vi "Chi-Squared (Non-Central) Moments.vi"(9 "d":dbl, 10 "k":i32=1) -> (0 "error":i32, 2 "variance":dbl=2.0, 3 "mean":dbl=1.0)   [LabVIEW 2014, in "NI_Gmath.lvlib"]
doc: "Returns the expected mean and variance of the random variate X, where X describes the selected distribution type. You must manually select the polymorphic instance to use."
uses:
  NI_Gmath.lvlib
  st_error_code.ctl
panel:
  # "Chi-Squared (Non-Central) Moments"
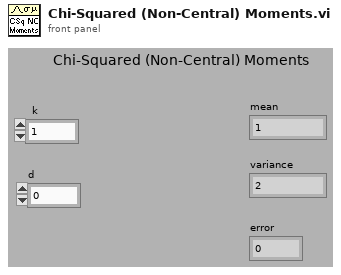
[diagram p1: front panel]
types:
  T1 = typedef "NI_Gmath.lvlib/st_error_code.ctl" = i32
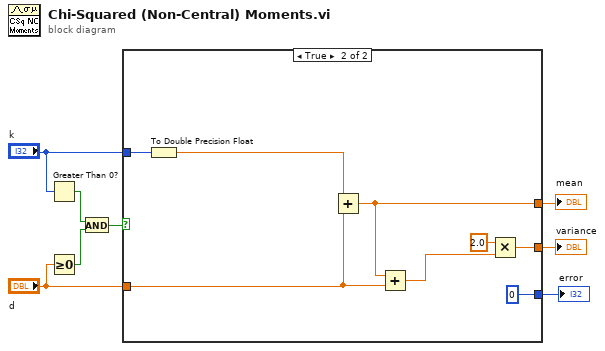
[diagram p0: block diagram]
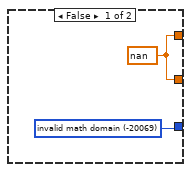
[diagram p2: hidden frame]
diagram:
  n1 = Greater Than 0?(x="k") -> (x > 0?=w8:bool)
  n2 = Greater Or Equal To 0?(x="d") -> (x >= 0?=w7:bool)
  n3 = And(x=w8, y=w7) -> (x .and. y?=w6:bool)
  n4 = case shown="True" w6 {
    tunnel: [w9 0 ("invalid math domain")] -> w3
    tunnel: [w10 w13] -> w5
    tunnel: "k" -> [_ w17]
    tunnel: [w10 w15] -> w4
    tunnel: "d" -> [_ w12]
    frame False {
      w9 = T1 -20069 items=["invalid math domain"=-20069, "Fourier interpolation size m >= n"=-20070, "empty array"=-20003] ("stat interp error code")
      w10 = nan
    }
    frame True {
      n5 = To Double Precision Float(number=w17) -> (double precision float=w14:dbl)
      n6 = Add(x=w14, y=w12) -> (x+y=w13:dbl)
      n7 = Add(x=w13, y=w12) -> (x+y=w11:dbl)
      n8 = Multiply(x=2.0, y=w11) -> (x*y=w15:dbl)
    }
  }
  "mean" <- w5
  "error" <- w3
  "variance" <- w4
